vi "DataTypeData.vi"(8 "error in (no error)":errorcluster, 9 "Data Type Names Array":string[](array[string]), 10 "ControlRefNums":refnum<vi>[](array[refnum]), 11 "FA Chosen Data Type":string) -> (0 "error out":errorcluster, 3 "ControlRefnumsArray":refnum<vi>[](array[refnum]))   [LabVIEW 2016, in "M1M3SupportEUI_Views.lvlib"]
uses:
  M1M3SupportEUI_Views.lvlib
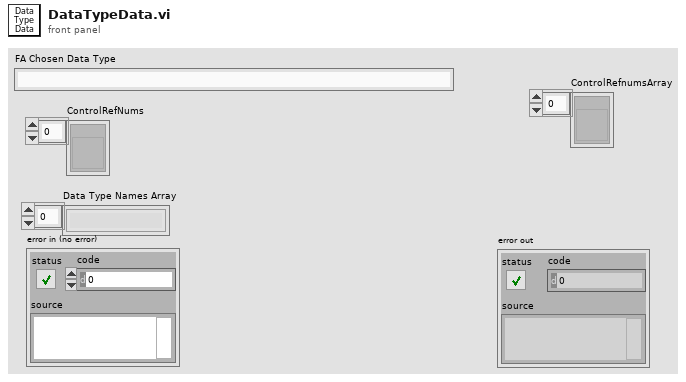
[diagram p1: front panel]
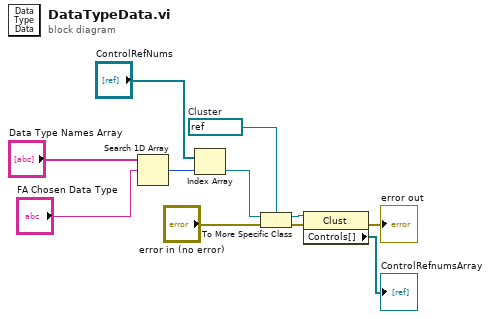
[diagram p0: block diagram]
diagram:
  w6 = refnum<vi> refnum  # Cluster
  n1 = Search 1D Array(1D array="Data Type Names Array", element="FA Chosen Data Type") -> (index of element=w8:i32)  [unwired: 1 in]
  n2 = Index Array(array="ControlRefNums", index=w8) -> (element=w7:refnum<vi>)
  n3 = To More Specific Class(target class=w6, reference=w7, error in="error in (no error)") -> (specific class reference=w5:refnum<vi>, error out=w4:errorcluster)
  n4 = property class="Clust"(reference=w5, error in=w4) -> (error out=→"error out":errorcluster, "Controls[]"=→"ControlRefnumsArray":refnum<vi>[])  [unwired: 1 out]
